vi "Robot Global Data.vi"() -> ()   [LabVIEW 2013]
doc: "This global VI can contain as many global variables as you need. Place a control on the panel, give it a good name. To read or write to it from a VI, drag the icon to the diagram of that VI. You can also drag from the project. Click on the node to change which global you access. You shouldn't have multiple locations writing to a global or it will cause a race-condition."
uses:
  <vilib>/Rock Robotics/WPI/Camera/WPI_CameraImageSize.ctl
  <vilib>/Rock Robotics/WPI/DriverStation/WPI_DriverStationRobotMode2.ctl
panel:
  out "KinectRUn?":bool
  out "KinectShoot?":bool
  in  "Encoder_Enum 2":enum16{"Reset", "Hold"}(ring)
  out "Left Drive Mult Out":dbl
  out "Right Drive Mult Out":dbl
  out "Drive Left Rate":dbl
  out "Drive Right Rate":dbl
  in  "Brake_Enum":enum16{"Reset", "Hold"}(ring)=enum."Hold"
  out "AutonCounter":dbl
  in  "Feeder_Enum":enum16{"Forward", "Back", "Stop"}(ring)=enum."Back"
  out "BACKLS":bool=TRUE
  out "FRONTLS":bool=TRUE
  out "AutoDriveR":dbl=-0.0
  out "AutoDriveL":dbl=-0.0
  out "SetFeeder":dbl
  out "RobotDistance":dbl
  out "ResetEncoders":bool
  out "Feeder Speed":dbl
  out "DSClimbD":bool
  out "DSFeederS":dbl
  out "DSFeederB":bool
  out "DSClutch":bool
  out "DSClimbU":bool
  out "DSClimb":bool
  out "DSFeederF":bool
  out "DSShoot":bool
  out "DSManual":bool=TRUE
  out "Feeder Addition":dbl
  in  "Wheels":bool
  in  "Feeder":bool
  in  "Encoder PID":bool
  out "DistanceEnable":dbl
  out "EncoderDistance":dbl
  out "Iterator":i32
  in  "Line Up":bool
  out "ArcadeEnabled":bool=TRUE
  out "Fly2Rate":dbl
  out "Fly1Rate":dbl
  out "Fly2":dbl
  out "Fly1":dbl
  out "Yaxis Signal":dbl
  out "Xaxis Addition":dbl
  in  "Line Up State":enum16{"Default", "Gyro", "Distance", "Shoot"}(ring)
  out "Center":dbl
  in  "Cluster 2":T1
  out "Zaxis":dbl
  out "Fly Wheel Multiplier":dbl
  out "Distance":dbl
  out "Fly Wheels Actual":dbl
  out "Fly Wheels Set":dbl
  out "Center Offset":dbl
  in  "image size":dbl
  out "Robot Angle":dbl
  out "Drive Right":dbl
  out "Drive Left":dbl
  out "Fly Wheel Back":i32
  out "Fly Wheel Front":i32
  out "Yaxis":dbl
  out "Xaxis":dbl
  in  "Robot Mode":T2
  in  "LED toggle rate (ms)":u32=20
  in  "image size":T3=enum."320x240"
  in  "Enable Vision":bool
  # "e"
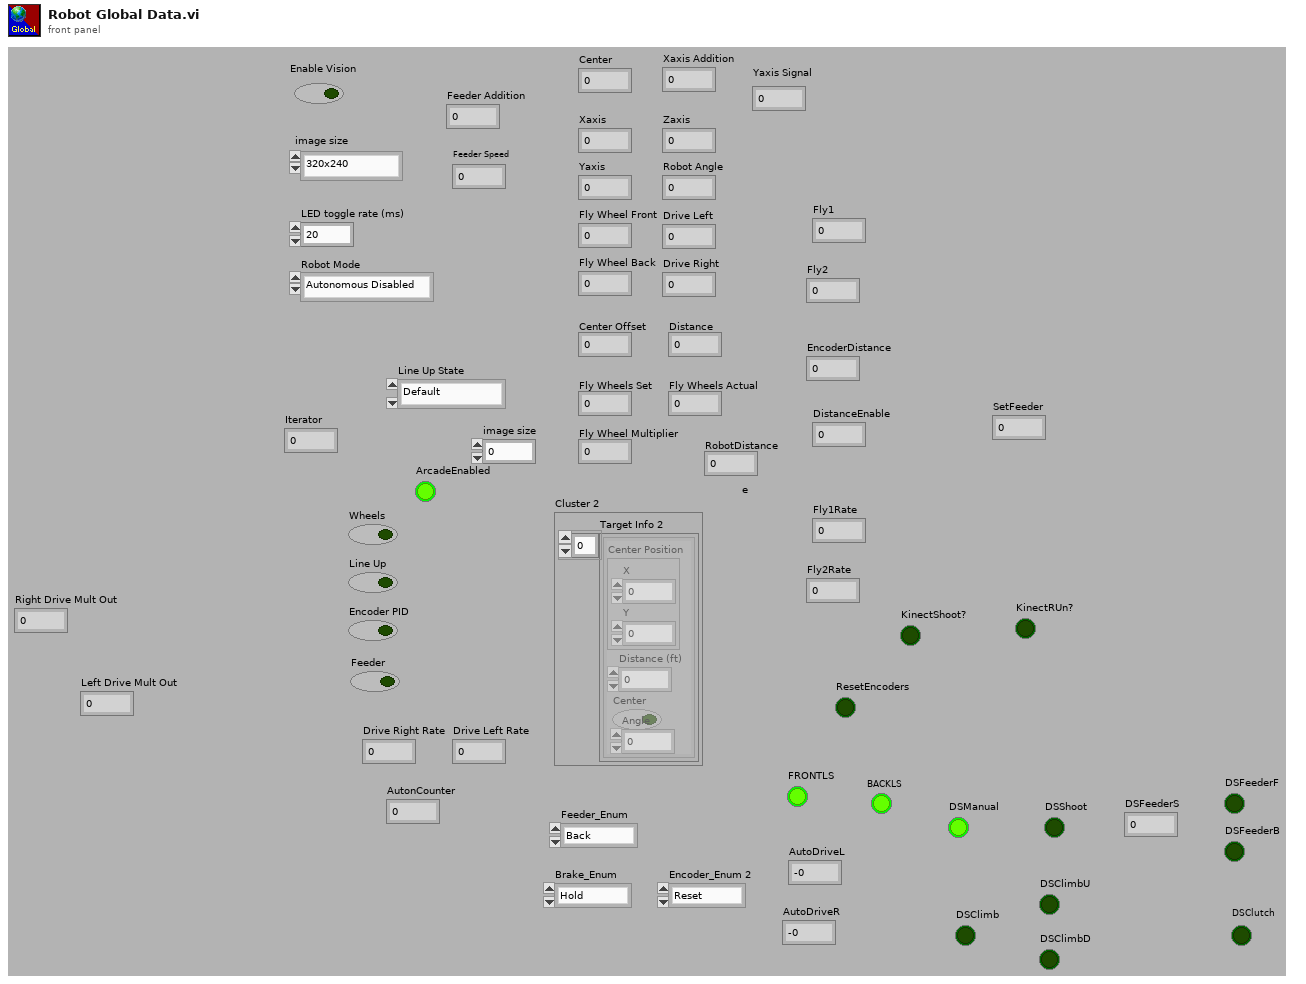
[diagram p1: front panel]
types:
  T1 = cluster{"Target Info 2":cluster{"Center Position":cluster{"X":dbl, "Y":dbl}, "Distance (ft)":dbl, "Center":bool, "Angle":dbl}[]}
  T2 = typedef "WPI_DriverStationRobotMode2.ctl" = enum16{"Autonomous Disabled", "Autonomous Enabled", "Teleop Disabled", "Teleop Enabled", "Timeout", "Finish", "Test Disabled", "Test Enabled"}
  T3 = typedef "WPI_CameraImageSize.ctl" = enum16{"640x480", "320x240", "160x120"}
diagram:
